vi "Are We Calibrating Actuator.vi"() -> ()   [LabVIEW 2012]
panel:
  out "Are We Calibrating Actuator?":bool
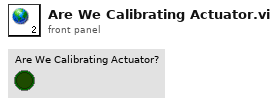
[diagram p1: front panel]
diagram:
